vi "curl POST JIRA Issue.vi"(7 "User Info (user:API Token)":string, 8 "error in (no error)":errorcluster, 9 "Create Issue Data":T1, 10 "Headers":T2[](array[typedef])=[{"Name"="Accept", "Content"="application/json"}, {"Name"="Content-Type", "Content"="application/json"}], 11 "Address":string) -> (0 "error out":errorcluster, 2 "return code":i32, 3 "Response":string)   [LabVIEW 2020]
doc: "Generates the cURL string to send to JIRA that will create a new issue with the information specified in the Create Issue Data. The address is the address in the form of \"https://your-domain.atlassian.net/rest/api/3/issue\" (with the quotes included). The Headers have been specified correctly for the version of the API that is current. The user name and API token need to be specified as user:API_Token.\n\nIssue Type in the Create Issue Data is specified as an ID number, how to do that for JIRA can be found that this URL: https://confluence.atlassian.com/jirakb/finding-the-id-for-issue-types-646186508.html\n\n12/2021 Choose Movement Consulting, LLC"
uses:
  JIRA_Header.ctl
  Create Issue Data.ctl
  Jira cURL text content.ctl
  Jira cURL paragarph content.ctl
  Jira cURL fields content.ctl
  <vilib>/addons/_JKI.lib/Serialization/JSON/JKI JSON Serialization.lvlib
panel:
  out "curl Command":string
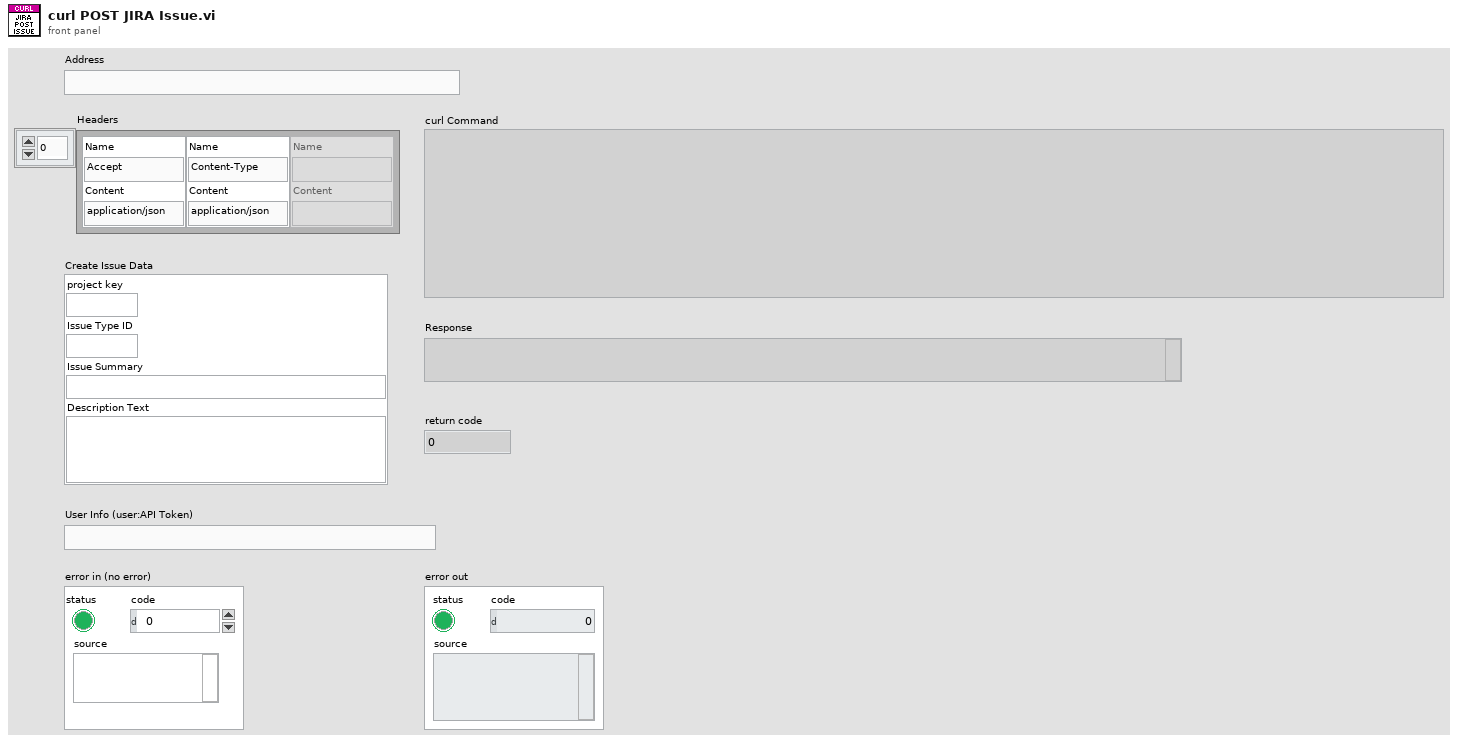
[diagram p1: front panel]
types:
  T1 = typedef "Create Issue Data.ctl" = cluster{"project key":string, "Issue Type ID":string, "Issue Summary":string, "Description Text":string}
  T2 = typedef "JIRA_Header.ctl" = cluster{"Name":string, "Content":string}
  T3 = typedef "Jira cURL fields content.ctl" = cluster{"issuetype":cluster{"id":string}, "project":cluster{"key":string}, "description":cluster{"version":i32, "type":string, "content":T4[]}, "summary":string}
  T4 = typedef "Jira cURL paragarph content.ctl" = cluster{"type":string, "content":T5[]}
  T5 = typedef "Jira cURL text content.ctl" = cluster{"type":string, "text":string}
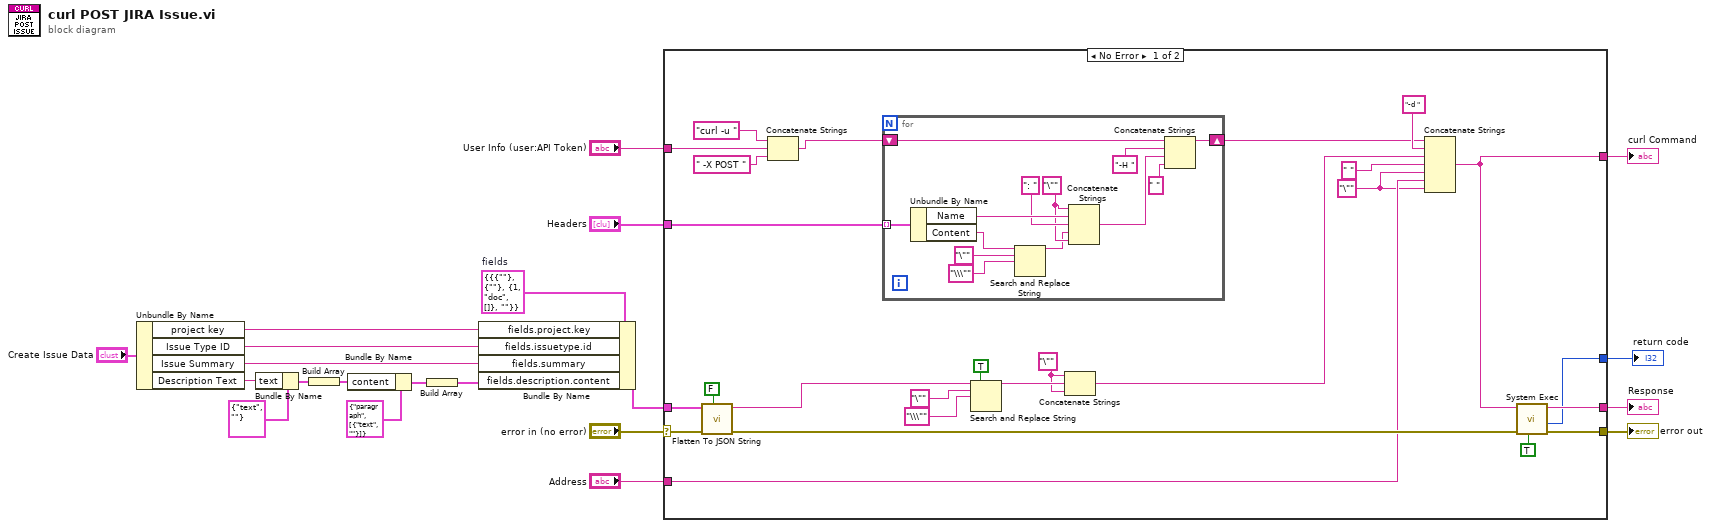
[diagram p0: block diagram]
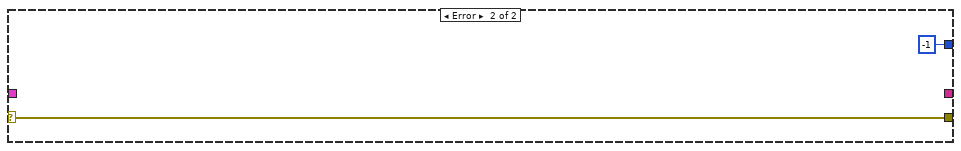
[diagram p2: hidden frame]
diagram:
  w1 = cluster{"fields":T3} {"fields"={"issuetype"={"id"=""}, "project"={"key"=""}, "description"={"version"=1, "type"="doc", "content"=[]}, "summary"=""}}  # fields
  n1 = Unbundle By Name("Create Issue Data") -> ("project key"=w13:string, "Issue Type ID"=w11:string, "Issue Summary"=w12:string, "Description Text"=w9:string)
  n2 = Bundle By Name(cluster=T5 {"type"="text", "text"=""} ("content"), "text"=w9) -> (w8:T5)
  n3 = Build Array(w8) -> (w5:T5[])
  n4 = Bundle By Name(cluster=T4 {"type"="paragraph", "content"=[{"type"="text", "text"=""}]} ("description content"), "content"=w5) -> (w7:T4)
  n5 = Build Array(w7) -> (w4:T4[])
  n6 = Bundle By Name(cluster=w1, "fields.project.key"=w13, "fields.issuetype.id"=w11, "fields.summary"=w12, "fields.description.content"=w4) -> (w15:cluster{"fields":T3})
  n7 = case shown="No Error" "error in (no error)" {
    selector: "error in (no error)" -> [w30 w62]
    tunnel: "Headers" -> [w47 _]
    tunnel: "Address" -> [w23 _]
    tunnel: [w36 _] -> w19
    tunnel: [w34 w62] -> w3
    tunnel: [w33 _] -> w18
    tunnel: "User Info (user:API Token)" -> [w29 _]
    tunnel: w15 -> [w25 _]
    tunnel: [w24 -1 ("return code")] -> w2
    frame No Error {
      w22 = "\"" ("string")
      w42 = "\""
      n8 = call <vilib>:"Flatten To JSON String.vi"("Multiline (T)"=FALSE, "error in (no error)"=w30, "Variant"=w25) -> ("error out"=w35:errorcluster, "JSON String"=w41:string)  [unwired: 7 in]
      n9 = Concatenate Strings("curl -u ", w29, " -X POST ") -> (w26:string)
      n10 = for {
        shift-right: [w48] -> w32
        shift-left: w26 -> [w49]
        tunnel: w47 -> [w60] mode=indexing
        w57 = "\""
        n11 = Unbundle By Name(w60) -> ("Name"=w59:string, "Content"=w55:string)
        n12 = Search and Replace String(input string=w55, search string="\"", replace string="\\\"" ("search string")) -> (result string=w56:string)  [unwired: 5 in, 3 out]
        n13 = Concatenate Strings(w57, w59, ": " ("string"), w56, w57) -> (w51:string)
        n14 = Concatenate Strings(w49, "-H " ("string"), w51, " " ("string")) -> (w48:string)
      }
      n15 = Search and Replace String(replace all?=TRUE ("replace all? (F)"), input string=w41, search string="\"", replace string="\\\"" ("search string")) -> (result string=w43:string)  [unwired: 4 in, 3 out]
      n16 = Concatenate Strings(w42, w43, w42) -> (w39:string)
      n17 = Concatenate Strings(w32, "-d " ("string"), w39, " " ("string"), w22, w23, w22) -> (w36:string)
      n18 = call <vilib>:"System Exec.vi"("run minimized? (F)"=TRUE, "error in (no error)"=w35, "command line"=w36) -> ("error out"=w34:errorcluster, "return code"=w24:i32, "standard output"=w33:string)  [unwired: 5 in, 1 out]
    }
    frame Error {
    }
  }
  "curl Command" <- w19
  "Response" <- w18
  "error out" <- w3
  "return code" <- w2
